vi "EnableDisable Switch.vi"(6 "?":bool, 8 "error in (no error)":errorcluster, 9 "True Disable":string[](array[string])=["", ""], 10 "True Enable":string[](array[string])=["", ""], 11 "CtlLookup Out":T1) -> (0 "error out":errorcluster, 3 "CtlLookup Out":T1)   [LabVIEW 2020, in "CtlReferences.lvlib" / "CtlReferences.lvclass"]
doc: "This VI will Enable/Disable the controls specified by name\nIf F is specified, the Arrays are swapped."
uses:
  CtlReferences.lvclass
  CtlReferences.lvclass/CtlReferences.ctl
  GetControlRef/GetControl_Control.vi
  TypeDefs/CtlLookup.ctl
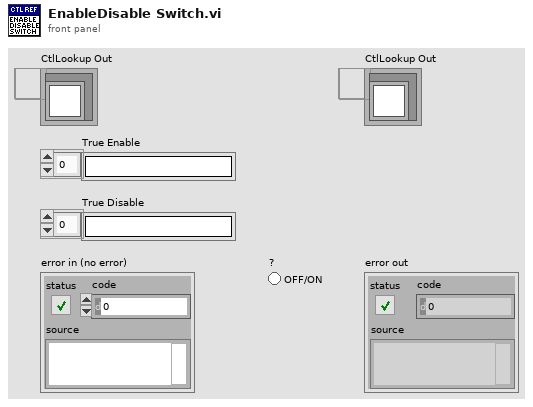
[diagram p1: front panel]
types:
  T1 = typedef "CtlReferences.lvlib/CtlReferences.lvclass/CtlLookup.ctl" = refnum<data-value>
  T2 = enum8{"Enabled", "Disabled", "Disabled and Grayed Out"}
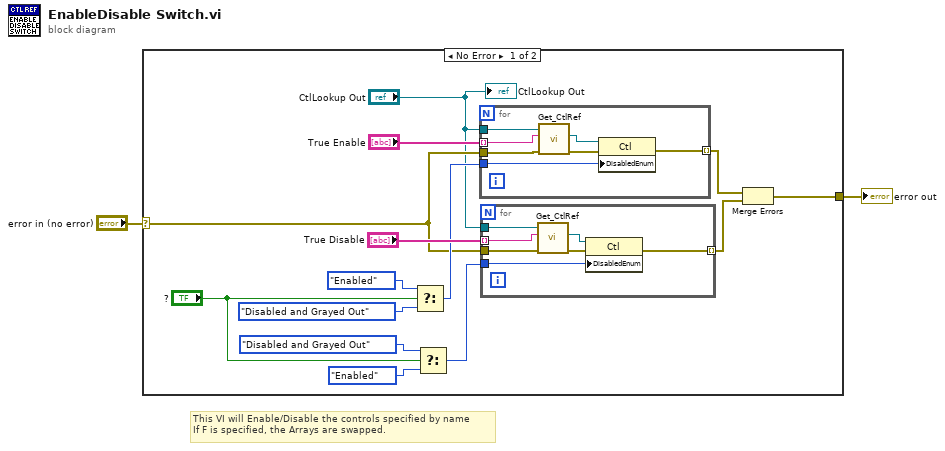
[diagram p0: block diagram]
diagram:
  # "This VI will Enable/Disable the controls specified by name\nIf F is specified, the Arrays are swapped."
  n1 = case shown="No Error" "error in (no error)" {
    selector: "error in (no error)" -> [w7 w31]
    tunnel: [w4 w31] -> w1
    frame No Error {
      n2 = Select(t=T2."Enabled" ("Disabled"), s="?", f=T2."Disabled and Grayed Out" ("Disabled")) -> (s? t:f=w10:T2)
      n3 = Select(t=T2."Disabled and Grayed Out" ("Disabled"), s="?", f=T2."Enabled" ("Disabled")) -> (s? t:f=w9:T2)
      n4 = for {
        tunnel: "CtlLookup Out" -> [w30]
        tunnel: "True Enable" -> [w29] mode=indexing
        tunnel: w10 -> [w26]
        tunnel: w7 -> [w25]
        tunnel: [w24] -> w6 mode=indexing
        n5 = call-poly "Get_CtlRef.vi"("error in (no error)"=w25, "Control Label"=w29, "CtlLookup In"=w30) -> ("error out"=w27:errorcluster, "Reference Out"=w28:refnum<vi>)  [unwired: 6 in, 1 out]
        n6 = property class="Ctl"(reference=w28, error in=w27, "DisabledEnum"=w26) -> (error out=w24:errorcluster)  [unwired: 1 out]
      }
      n7 = for {
        tunnel: "CtlLookup Out" -> [w23]
        tunnel: "True Disable" -> [w22] mode=indexing
        tunnel: w9 -> [w19]
        tunnel: w7 -> [w18]
        tunnel: [w17] -> w5 mode=indexing
        n8 = call-poly "Get_CtlRef.vi"("error in (no error)"=w18, "Control Label"=w22, "CtlLookup In"=w23) -> ("error out"=w21:errorcluster, "Reference Out"=w20:refnum<vi>)  [unwired: 6 in, 1 out]
        n9 = property class="Ctl"(reference=w20, error in=w21, "DisabledEnum"=w19) -> (error out=w17:errorcluster)  [unwired: 1 out]
      }
      n10 = Merge Errors(w6, w5) -> (w4:errorcluster)
      "CtlLookup Out" <- "CtlLookup Out"
    }
    frame Error {
    }
  }
  "error out" <- w1
